vi "FA_AddOrderToConfigData.vi"(11 "Config in":T1) -> (3 "Config":T1)   [LabVIEW 2014, in "FA_NativeTypes.lvlib"]
doc: "Prepends the array index to each name in the parameter array"
uses:
  FA_NativeTypes.lvlib
  FA_Config.ctl
  FA_LocalStore API/source/VI Source/FA_LSSpecialTypes.ctl
  FA_LocalStore API/source/VI Source/FA_LocalStore.lvlib
panel:
  out "Error Out":errorcluster
  in  "Error In":errorcluster
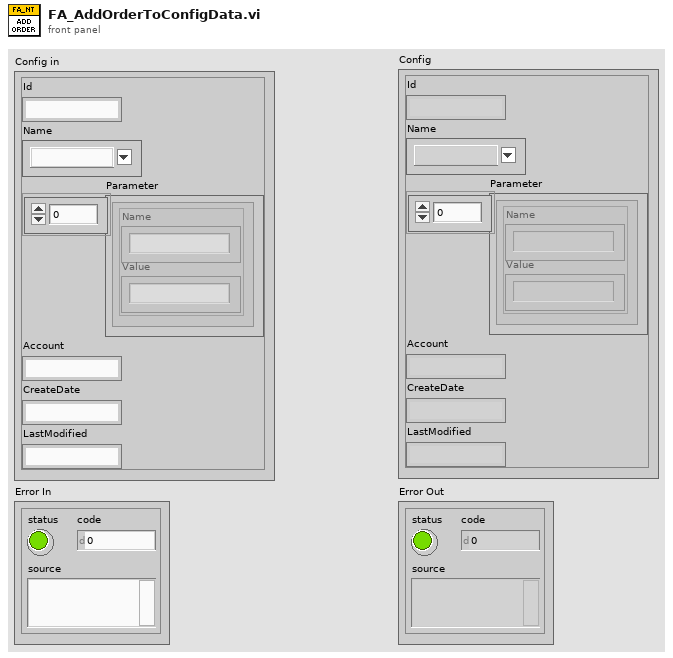
[diagram p1: front panel]
types:
  T1 = typedef "FA_NativeTypes.lvlib/FA_Config.ctl" = cluster{"Id":string, "Name":T2, "Parameter":cluster{"Name":string, "Value":string}[], "Account":string, "CreateDate":string, "LastModified":string}
  T2 = typedef "FA_LocalStore.lvlib/FA_LSSpecialTypes.ctl" = string
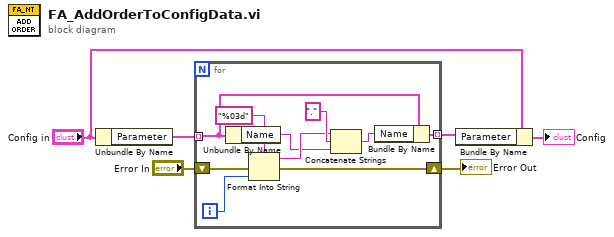
[diagram p0: block diagram]
diagram:
  n1 = Unbundle By Name("Config in") -> ("Parameter"=w3:cluster{"Name":string, "Value":string}[])
  n2 = for {
    tunnel: w3 -> [w16] mode=indexing
    tunnel: [w15] -> w4 mode=indexing
    shift-right: [w12] -> w1
    shift-left: "Error In" -> [w13]
    i -> [w14]
    n3 = Unbundle By Name(w16) -> ("Name"=w8:string)
    n4 = Format Into String(format string="%03d", error in=w13, w14) -> (resulting string=w9:string, error out=w12:errorcluster)  [unwired: 1 in]
    n5 = Concatenate Strings(w9, "." ("string"), w8) -> (w10:string)
    n6 = Bundle By Name(cluster=w16, "Name"=w10) -> (w15:cluster{"Name":string, "Value":string})
  }
  "Error Out" <- w1
  n7 = Bundle By Name(cluster="Config in", "Parameter"=w4) -> (→"Config":T1)
